vi "Colouring.vi"(11 "Lighting Mode":T1) -> (3 "Colors [4]":cluster{"Numeric":u32, "Numeric":u32}[](array[cluster]))   [LabVIEW 2021]
uses:
  Type defs/Lighting Modes.ctl
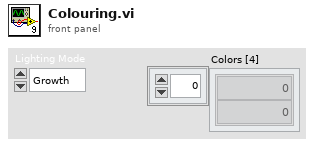
[diagram p1: front panel]
types:
  T1 = typedef "Lighting Modes.ctl" = enum16{"Growth", "Harvest", "Night"}
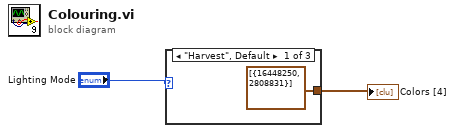
[diagram p0: block diagram]
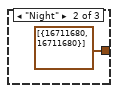
[diagram p2: hidden frame]
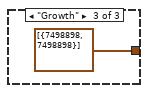
[diagram p3: hidden frame]
diagram:
  n1 = case shown="\"Harvest\", Default" "Lighting Mode" {
    tunnel: [cluster{u32, u32}[] [{16448250, 2808831}] ("Colors [4]") cluster{u32, u32}[] [{16711680, 16711680}] ("Colors [4]") cluster{u32, u32}[] [{7498898, 7498898}] ("Colors [4]")] -> w1
    frame "Harvest", Default {
    }
    frame "Night" {
    }
    frame "Growth" {
    }
  }
  "Colors [4]" <- w1
